vi "ConfigureVirtualChannels.vi"(6 "not supported virtual channels":string[](array[string]), 7 "DisableDeviceAnalysis":bool, 8 "error in (no error)":errorcluster, 9 "settling time (seconds)":dbl, 10 "data group name":string, 11 "channels in this group":T1[](array[typedef])) -> (0 "error out":errorcluster, 1 "atleast one virtual channel":bool, 3 "virtual channel config":T4)   [LabVIEW 2017, in "CmsVirtualChannel.lvlib"]
uses:
  <vilib>/addons/InsightCM/Devices/Shared/Cms/CmsVirtualChannel/CmsVirtualChannel.lvlib
  <vilib>/addons/InsightCM/Devices/Shared/Cms/CmsVirtualChannel/controls/VirtualChannelGroup.ctl
  <vilib>/addons/InsightCM/Devices/Shared/Cms/CmsVirtualChannel/controls/VirtualChannel.ctl
  <vilib>/addons/InsightCM/MessageBus/Base/controls/R2_Channel.ctl
  <vilib>/addons/InsightCM/MessageBus/Base/controls/KeyValuePair.ctl
  <vilib>/addons/InsightCM/MessageBus/Base/controls/Metric.ctl
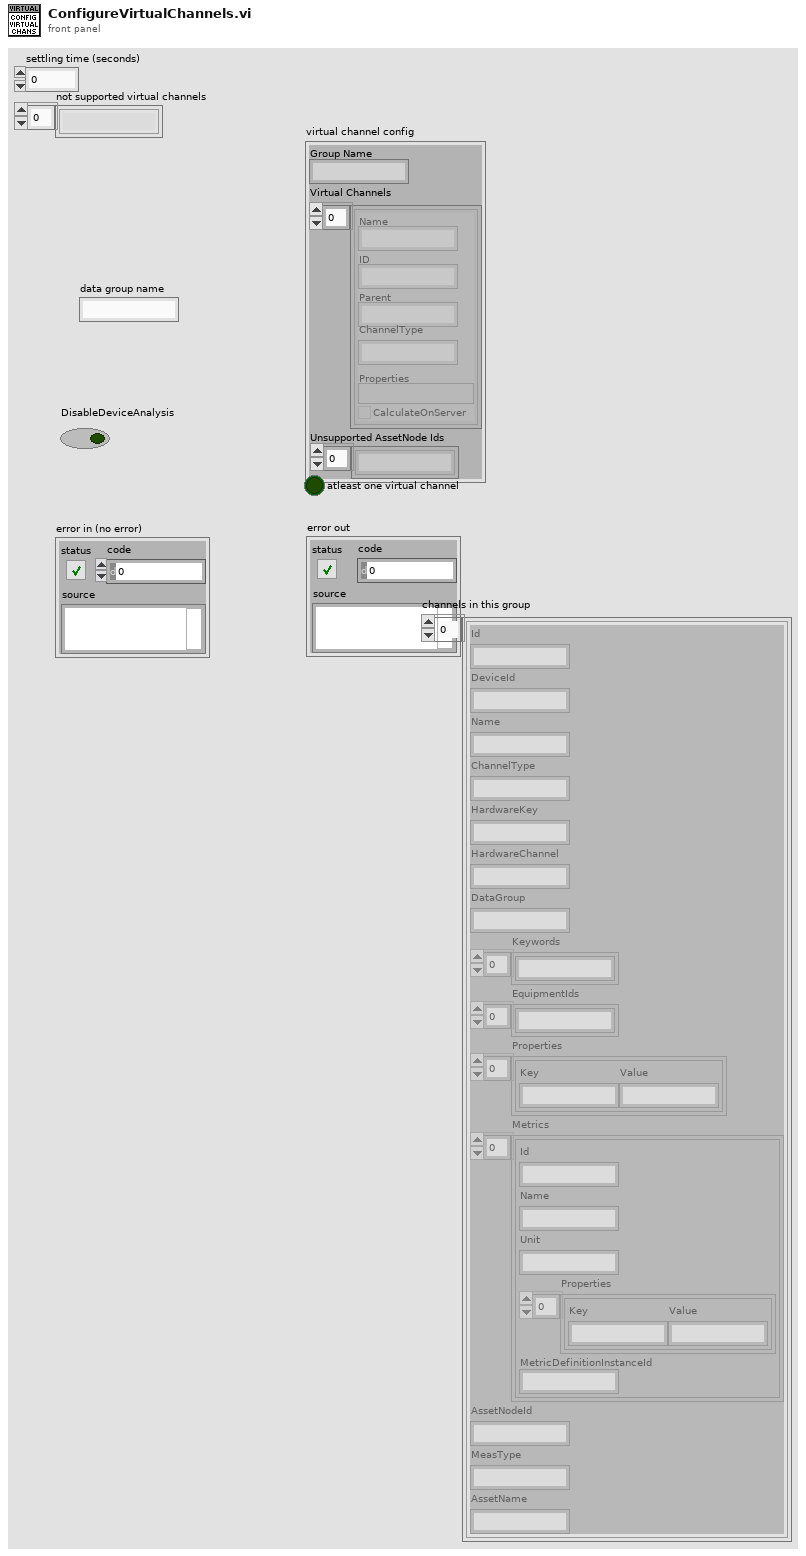
[diagram p1: front panel]
types:
  T1 = typedef "R2_Channel.ctl" = cluster{"Id":string, "DeviceId":string, "Name":string, "ChannelType":string, "HardwareKey":string, "HardwareChannel":string, "DataGroup":string, "Keywords":string[], "EquipmentIds":string[], "Properties":T2[], "Metrics":T3[], "AssetNodeId":string, "MeasType":string, "AssetName":string}
  T2 = typedef "KeyValuePair.ctl" = cluster{"Key":string, "Value":string}
  T3 = typedef "Metric.ctl" = cluster{"Id":string, "Name":string, "Unit":string, "Properties":T2[], "MetricDefinitionInstanceId":string}
  T4 = typedef "CmsVirtualChannel.lvlib/VirtualChannelGroup.ctl" = cluster{"Group Name":string, "Virtual Channels":T5[], "Unsupported AssetNode Ids":string[]}
  T5 = typedef "CmsVirtualChannel.lvlib/VirtualChannel.ctl" = cluster{"Name":string, "ID":string, "Parent":string, "ChannelType":string, "Properties":variant, "CalculateOnServer":bool}
  T6 = typedef "CmsVirtualChannel.lvlib/Tachometer.ctl" = cluster{"Tachometer Slope":string, "Pulses Per Rev":i32, "Tachometer Threshold":dbl, "Tachometer Hysteresis":dbl, "Sensitivity":dbl, "Type":string, "Tach State":T7, "Settling Time":dbl}
  T7 = typedef "VibrationAnalysisFunctions.lvlib/Tachometer.ctl" = cluster{"Reset":bool, "analog tach state":cluster{"last value":dbl, "edge state":cluster{"processed data":dbl, "buffer data":dbl[]}}, "digital tach state in":T8, "speed state":cluster{"state":enum16{"0 Pulses", "1 Pulse", "2+ Pulses"}, "last pulse position":dbl, "RPM":dbl, "Empty Blocks":i32}}
  T8 = typedef "VibrationAnalysisFunctions.lvlib/DigitalTachometer.ctl" = cluster{dbl[], i32, "not enough pulses?":bool, "pulse buffer out":dbl[], i32, "final state":dbl[], "duration":dbl, "reset":bool, "overflow state":cluster{"low speed state":cluster{dbl, ext}, "counter state":cluster{"counter task type":enum16{"period measurement", "event counting"}, "t":dbl, "t":dbl}}, "OS Clk Start":dbl}
  T9 = typedef "CmsVirtualChannel.lvlib/Integration.ctl" = cluster{"Conversion Op":T10, "Unit":string, "Parent Unit":string, "Single Integration Cutoff":dbl, "Double Integration Cutoff":dbl, "Lowpass Filter State":T11, "Highpass Filter State":T12, "Wfm Scale":sgl}
  T10 = typedef "AnalysisHelper.lvlib/ConversionOp.ctl" = enum16{"none", "singleInt", "doubleInt", "singleDiff", "doubleDiff"}
  T11 = typedef "VibrationAnalysisFunctions.lvlib/LowPassFilterState.ctl" = cluster{"designed":bool, "integration filter coefficients":cluster{"beta":dbl, "gamma":dbl, "alpha":dbl}, "state":cluster{"x(n-1) state":dbl, "y(n-1) state":dbl, "x(n-2) state":dbl, "y(n-2) state":dbl}}
  T12 = typedef "VibrationAnalysisFunctions.lvlib/HighPassFilterState.ctl" = cluster{"designed":bool, "IIR Filter Cluster":cluster{"filter structure":enum32{"IIR 2nd Order", "IIR 4th Order"}, "Reverse Coefficients":dbl[], "Forward Coefficients":dbl[]}, "Filter State":dbl[]}
  T13 = typedef "CmsVirtualChannel.lvlib/Differentiation.ctl" = cluster{"Conversion Op":T10, "Unit":string, "Parent Unit":string}
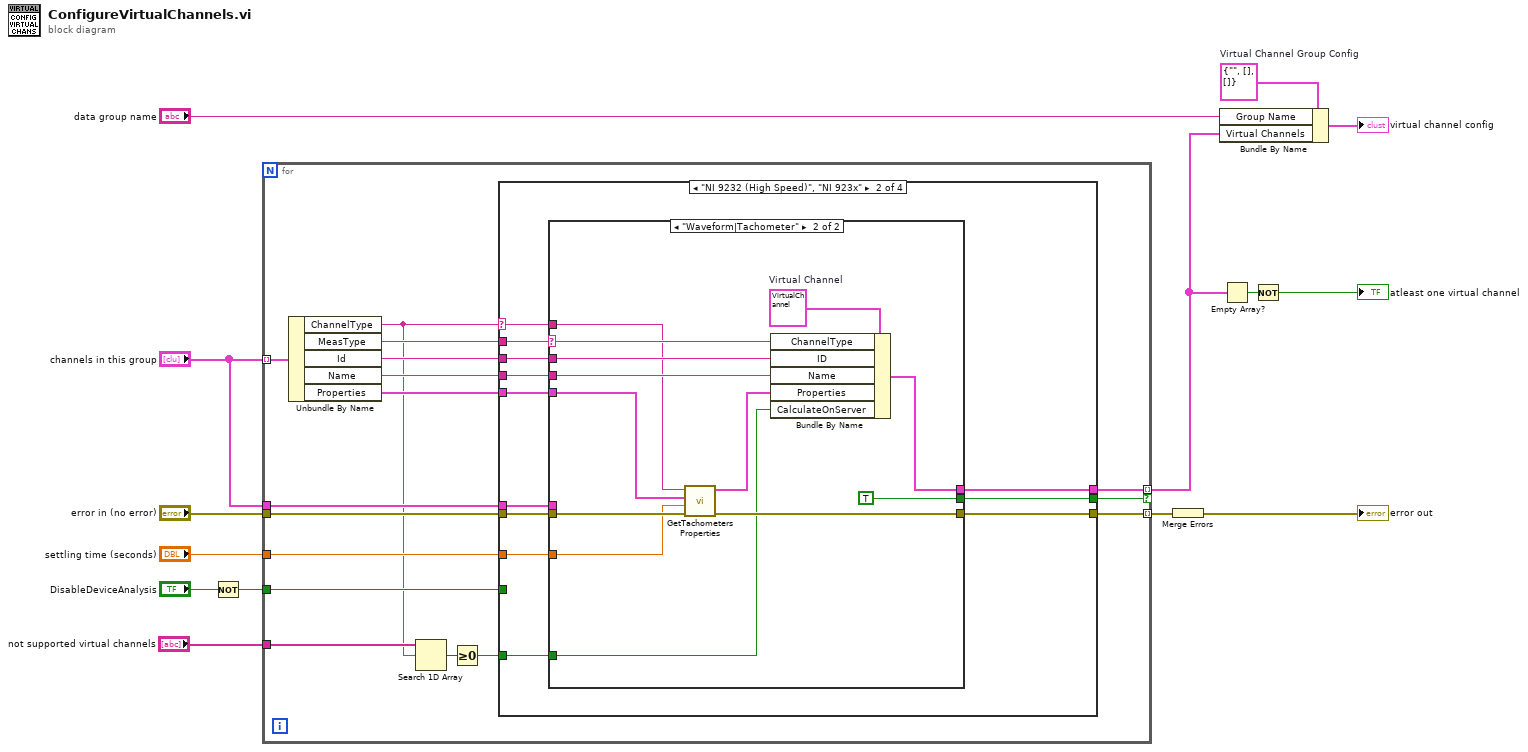
[diagram p0: block diagram]
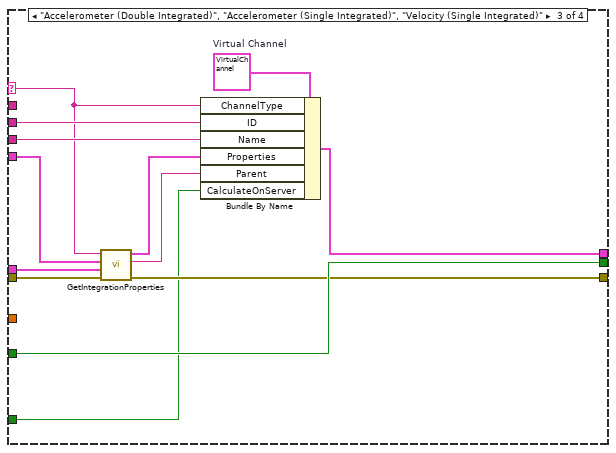
[diagram p4: hidden frame]
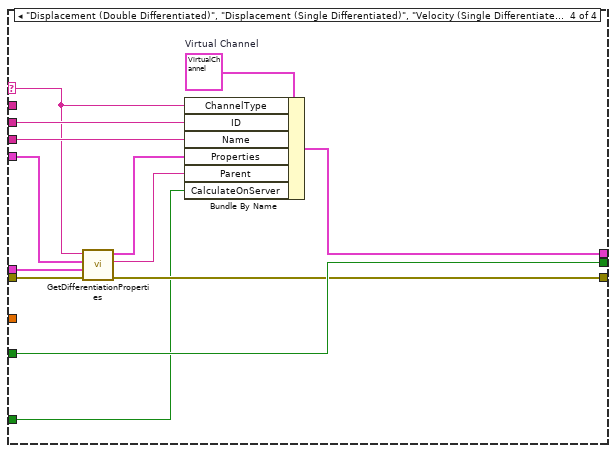
[diagram p5: hidden frame]
diagram:
  w13 = T4 {"Group Name"="", "Virtual Channels"=[], "Unsupported AssetNode Ids"=[]}  # Virtual Channel Group Config
  n1 = Not(x="DisableDeviceAnalysis") -> (.not. x?=w5:bool)
  n2 = for {
    tunnel: "channels in this group" -> [w30] mode=indexing
    tunnel: [w28] -> w10 mode=indexing if=w27
    tunnel: "error in (no error)" -> [w26]
    tunnel: [w25] -> w3 mode=indexing
    tunnel: "channels in this group" -> [w23]
    tunnel: w5 -> [w21]
    tunnel: "settling time (seconds)" -> [w19]
    tunnel: "not supported virtual channels" -> [w18]
    n3 = Unbundle By Name(w30) -> ("ChannelType"=w17:string, "MeasType"=w20:string, "Id"=w22:string, "Name"=w29:string, "Properties"=w24:T2[])
    n4 = Search 1D Array(1D array=w18, element=w17) -> (index of element=w16:i32)  [unwired: 1 in]
    n5 = Greater Or Equal To 0?(x=w16) -> (x >= 0?=w15:bool)
    n6 = case shown="\"NI 9232 (High Speed)\", \"NI 923x\"" w17 {
      selector: w17 -> [_ w33 w65 w78]
      tunnel: w24 -> [_ w37 w64 w77]
      tunnel: w29 -> [_ w41 w67 w80]
      tunnel: [_ w38 w58 w71] -> w28
      tunnel: w26 -> [_ w40 w60 w75]
      tunnel: [_ w39 w59 w74] -> w25
      tunnel: [_ w35 w66 w79] -> w27
      tunnel: w22 -> [_ w42 w68 w81]
      tunnel: w23 -> [_ w36 w63 w76]
      tunnel: w21 -> [_ _ w66 w79]
      tunnel: w20 -> [_ w34 _ _]
      tunnel: w19 -> [_ w32 _ _]
      tunnel: w15 -> [_ w31 w57 w70]
      frame Default {
      }
      frame "NI 9232 (High Speed)", "NI 923x" {
        n7 = case shown="\"Waveform|Tachometer\"" w34 {
          selector: w34 -> [_ w47]
          tunnel: w42 -> [_ w55]
          tunnel: w41 -> [_ w54]
          tunnel: w40 -> [w43 w51]
          tunnel: [w43 w49] -> w39
          tunnel: [_ w48] -> w38
          tunnel: w37 -> [_ w52]
          tunnel: w36 -> [_ _]
          tunnel: [_ TRUE] -> w35
          tunnel: w33 -> [_ w46]
          tunnel: w32 -> [_ w45]
          tunnel: w31 -> [_ w44]
          frame Default {
          }
          frame "Waveform|Tachometer" {
            w56 = T5 {"Name"="", "ID"="", "Parent"="", "ChannelType"="", "Properties"=variant(cluster{"Key":string, "Value":string}[] []), "CalculateOnServer"=FALSE}  # Virtual Channel
            n8 = call <vilib>:"GetTachometersProperties.vi"("error in (no error)"=w51, "settling time (seconds)"=w45, "channel properties"=w52, "channel type"=w46) -> ("error out"=w49:errorcluster, "tachometer"=w50:T6)  [unwired: 6 in]
            n9 = Bundle By Name(cluster=w56, "ChannelType"=w47, "ID"=w55, "Name"=w54, "Properties"=w50, "CalculateOnServer"=w44) -> (w48:T5)
          }
        }
      }
      frame "Accelerometer (Double Integrated)", "Accelerometer (Single Integrated)", "Velocity (Single Integrated)" {
        w69 = T5 {"Name"="", "ID"="", "Parent"="", "ChannelType"="", "Properties"=variant(cluster{"Key":string, "Value":string}[] []), "CalculateOnServer"=FALSE}  # Virtual Channel
        n10 = call <vilib>:"GetIntegrationProperties.vi"("error in (no error)"=w60, "Channels"=w63, "Channel Properties"=w64, "ChannelType"=w65) -> ("error out"=w59:errorcluster, "Parent Channel Name"=w62:string, "Integration Properties"=w61:T9)  [unwired: 5 in]
        n11 = Bundle By Name(cluster=w69, "ChannelType"=w65, "ID"=w68, "Name"=w67, "Properties"=w61, "Parent"=w62, "CalculateOnServer"=w57) -> (w58:T5)
      }
      frame "Displacement (Double Differentiated)", "Displacement (Single Differentiated)", "Velocity (Single Differentiated)" {
        w82 = T5 {"Name"="", "ID"="", "Parent"="", "ChannelType"="", "Properties"=variant(cluster{"Key":string, "Value":string}[] []), "CalculateOnServer"=FALSE}  # Virtual Channel
        n12 = call <vilib>:"GetDifferentiationProperties.vi"("error in (no error)"=w75, "Channels"=w76, "Channel Properties"=w77, "ChannelType"=w78) -> ("error out"=w74:errorcluster, "Parent Channel Name"=w73:string, "Differentiation Properties"=w72:T13)  [unwired: 5 in]
        n13 = Bundle By Name(cluster=w82, "ChannelType"=w78, "ID"=w81, "Name"=w80, "Properties"=w72, "Parent"=w73, "CalculateOnServer"=w70) -> (w71:T5)
      }
    }
  }
  n14 = Merge Errors(w3) -> (→"error out":errorcluster)
  n15 = Bundle By Name(cluster=w13, "Group Name"="data group name", "Virtual Channels"=w10) -> (→"virtual channel config":T4)
  n16 = Empty Array?(array=w10) -> (empty?=w9:bool)
  n17 = Not(x=w9) -> (.not. x?=→"atleast one virtual channel":bool)
